vi "MS IRISS V2.vi"(8 "Stage Cmd Posit":dbl[](array[numeric])=[0.0, 0.0, 0.0], 9 "L5 cmd Posit":dbl, 10 "Joint Cmd Posit":dbl[](array[numeric]), 11 "ArmID":i32) -> (0 "Stage Out Posit":dbl[](array[numeric]), 1 "L5 Out Posit":dbl, 2 "Joint Out Posit":dbl[](array[numeric]), 3 "Connection Status":bool, 4 "Receive Count":u64, 6 "Send Count":u64)   [LabVIEW 2016]
uses:
  Subsystems/Global Variables.vi
panel:
  in  "XYZ Control or Joint Control":bool
  in  "E-STOP button":bool caption="Stop Button"
  in  "Tooltip XYZ Cmd":T1={"x"=0.0, "y"=0.0, "z"=-10.0, "roll"=0.0, "grasp"=0.0}
  in  "Stop Labview Button":bool caption="Stop Button"
  out "Tooltip XYZ Out":T1
  # "Robot Status"
  # "Robot XYZ Command (kinematics included)"
  # "Joint Angle Command (for debug and testing)"
  # "For debug only, No need to use this button during labview operation, if does, then the low level control will be terminated, and everything will have to be rerestarted including homing"
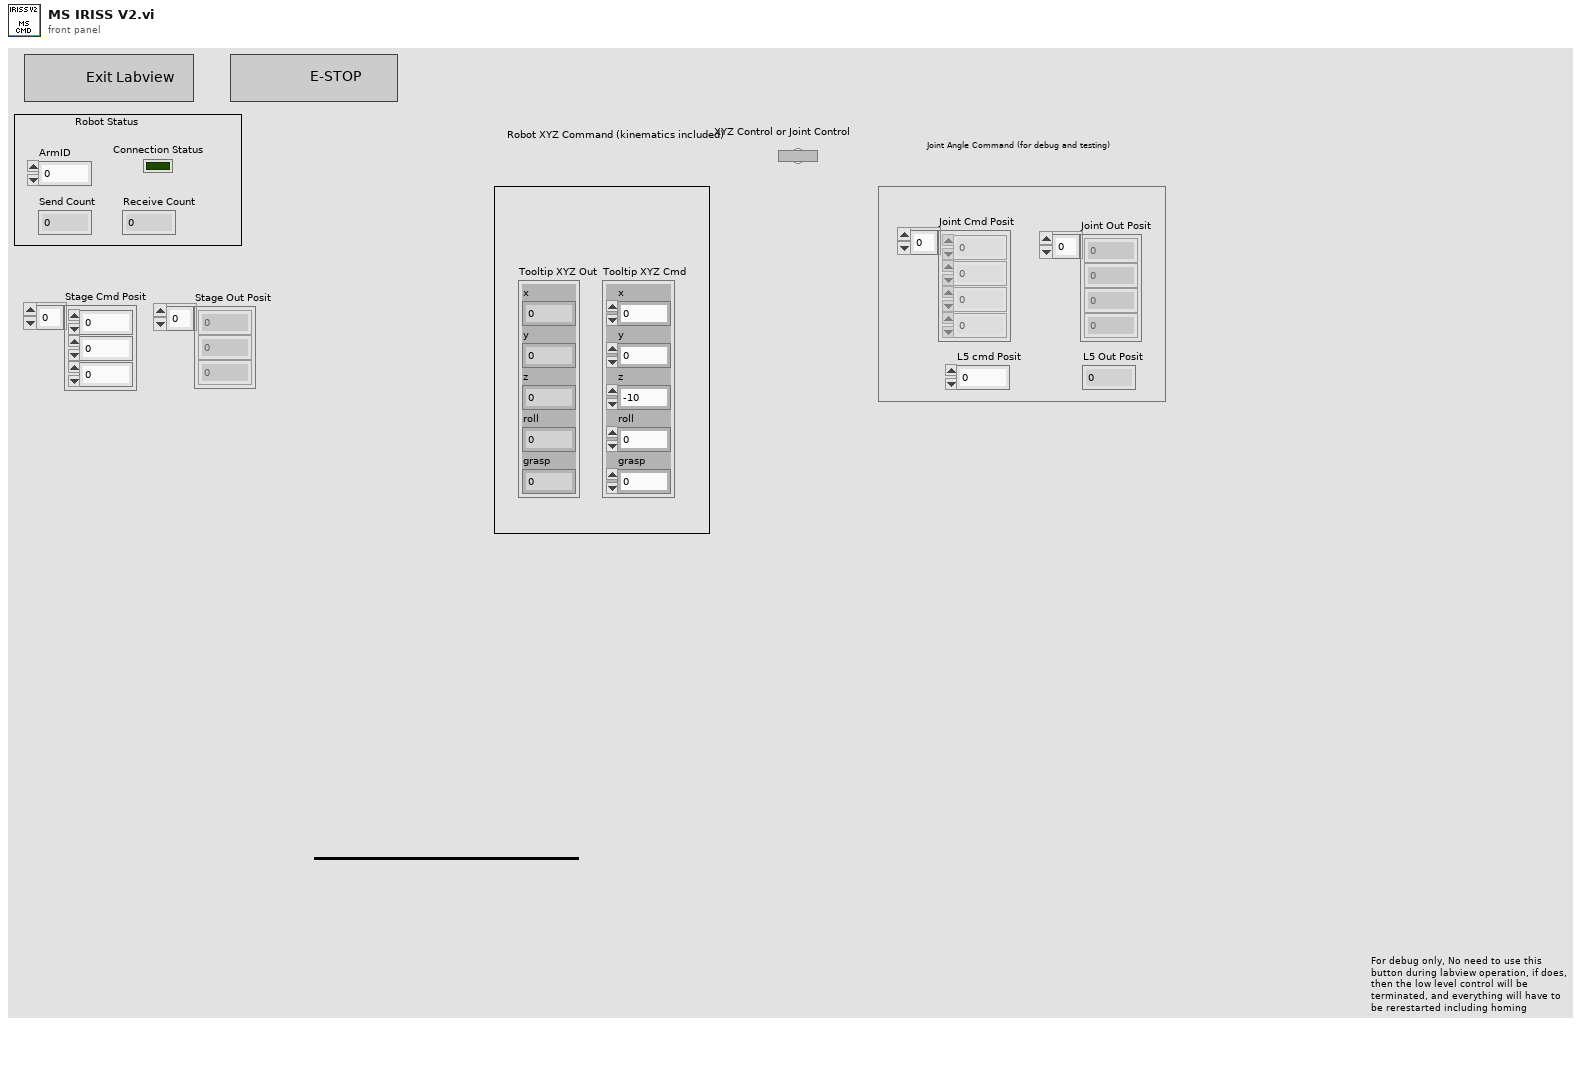
[diagram p1: front panel]
types:
  T1 = cluster{"x":dbl, "y":dbl, "z":dbl, "roll":dbl, "grasp":dbl}
  T2 = cluster{"StagePosition - X":dbl, "StagePosition - X":dbl, "StagePosition - X":dbl, "StagePosition - X":dbl, "L5 cmd Posit":dbl, "StagePosition - X":dbl, "StagePosition - X":dbl, "StagePosition - X":dbl}
  T3 = cluster{"j0":dbl, "j1":dbl, "j2":dbl, "j3":dbl, "j4":dbl, "j5":dbl, "j6":dbl, "j7":dbl}
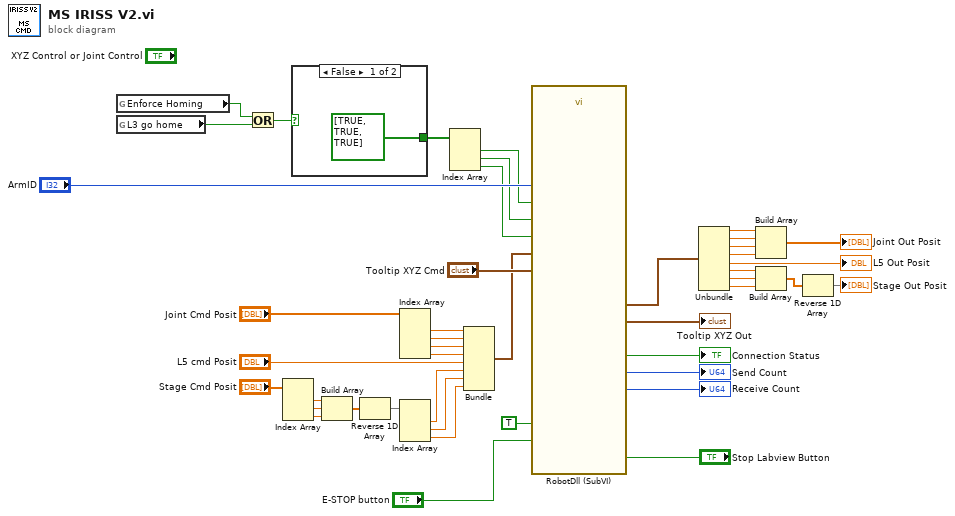
[diagram p0: block diagram]
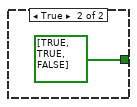
[diagram p2: hidden frame]
diagram:
  n1 = global read "Global Variables.vi" "Enforce Homing"() -> (w11:bool)
  n2 = global read "Global Variables.vi" "L3 go home"() -> (w6:bool)
  n3 = Or(x=w11, y=w6) -> (x .or. y?=w12:bool)
  n4 = Index Array(array="Stage Cmd Posit") -> (element #1=w4:dbl, element #2=w3:dbl, element #3=w2:dbl)  [unwired: 3 in]
  n5 = case shown="False" w12 {
    tunnel: [bool[] [TRUE, TRUE, TRUE] bool[] [TRUE, TRUE, FALSE]] -> w15
    frame False {
    }
    frame True {
    }
  }
  n6 = Build Array(w4, w3, w2) -> (w1:dbl[])
  n7 = Reverse 1D Array(array=w1) -> (reversed array=w10:dbl[])
  n8 = Index Array(array="Joint Cmd Posit") -> (element #1=w35:dbl, element #2=w34:dbl, element #3=w33:dbl, element #4=w32:dbl)  [unwired: 4 in]
  n9 = Index Array(array=w10) -> (element #1=w31:dbl, element #2=w30:dbl, element #3=w29:dbl)  [unwired: 3 in]
  n10 = Index Array(array=w15) -> (element #1=w16:bool, element #2=w14:bool, element #3=w13:bool)  [unwired: 3 in]
  n11 = Bundle("StagePosition - X"=w35, "StagePosition - X"=w34, "StagePosition - X"=w33, "StagePosition - X"=w32, "L5 cmd Posit"="L5 cmd Posit", "StagePosition - X"=w31, "StagePosition - X"=w30, "StagePosition - X"=w29) -> (w28:T2)  [unwired: 1 in]
  n12 = call "RobotDll (SubVI).vi"("ArmPower"=w16, "Control Mode"=TRUE ("XYZ Control or Joint Control"), "XYZ Stage Power"=w14, "E-STOP button"="E-STOP button", "robot xyz command"="Tooltip XYZ Cmd", "ArmID"="ArmID", "Run"=w13, "Stop Button in"="Stop Labview Button", "joint command"=w28) -> ("Tooltip"=→"Tooltip XYZ Out":T1, "ReceiveCount"=→"Receive Count":u64, "ActualJointAngles"=w26:T3, "SendCount"=→"Send Count":u64, "RobotConnection"=→"Connection Status":bool)  [unwired: 4 in, 2 out]
  n13 = Unbundle(w26) -> ("j0"=w25:dbl, "j1"=w24:dbl, "j2"=w23:dbl, "j3"=w22:dbl, "j4"=→"L5 Out Posit":dbl, "j5"=w20:dbl, "j6"=w19:dbl, "j7"=w18:dbl)
  n14 = Build Array(w25, w24, w23, w22) -> (→"Joint Out Posit":dbl[])
  n15 = Build Array(w20, w19, w18) -> (w9:dbl[])
  n16 = Reverse 1D Array(array=w9) -> (reversed array=→"Stage Out Posit":dbl[])
